vi "Load.vi"(0 "DashboardServer in":refnum<class "Dashboard Server.lvclass">, 1 "program":string, 5 "error in (no error)":errorcluster) -> (14 "DashboardServer out":refnum<class "Dashboard Server.lvclass">, 15 "returnStatus":string, 19 "error out":errorcluster)   [LabVIEW 2016, in "Dashboard Server.lvclass"]
uses:
  Dashboard Server.lvclass
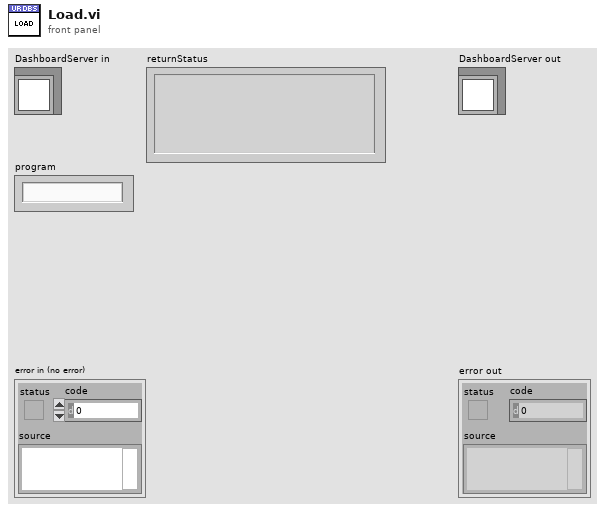
[diagram p1: front panel]
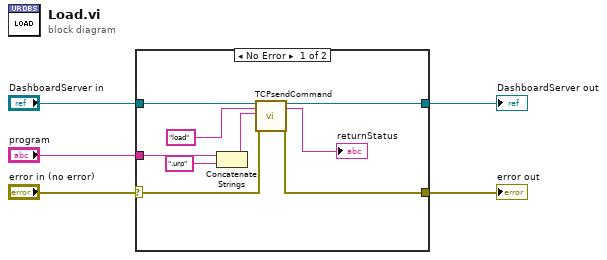
[diagram p0: block diagram]
diagram:
  n1 = case shown="No Error" "error in (no error)" {
    selector: "error in (no error)" -> [w12 w16]
    tunnel: [w11 w16] -> w4
    tunnel: [w13 w15] -> w2
    tunnel: "DashboardServer in" -> [w14 w15]
    tunnel: "program" -> [w8 _]
    frame No Error {
      n2 = Concatenate Strings(w8, ".urp" ("string")) -> (w7:string)
      n3 = call-dynamic "TCPsendCommand.vi"("DashboardServer in"=w14, "command"="load", "data"=w7, "error in (no error)"=w12) -> ("DashboardServer out"=w13:refnum<class "Dashboard Server.lvclass">, "returnStatus"=→"returnStatus":string, "error out"=w11:errorcluster)  [unwired: 12 in, 1 out]
    }
    frame Error {
    }
  }
  "error out" <- w4
  "DashboardServer out" <- w2
